vi "Configure Alarm.vi"(8 "error in (no error)":errorcluster, 10 "Alarm Clear Method (0: Safe)":i32(ring) items=["Safe", "Auto"], 11 "VISA resource name":refnum<visa-resource-name>) -> (0 "error out":errorcluster, 3 "VISA resource name out":refnum<visa-resource-name>)   [LabVIEW 2023]
doc: "Configures the method of clearing OHP, FAN, AC-FAIL, and SD alarms."
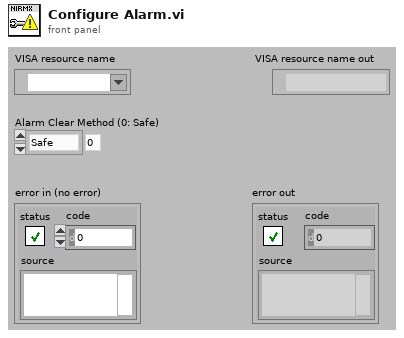
[diagram p1: front panel]
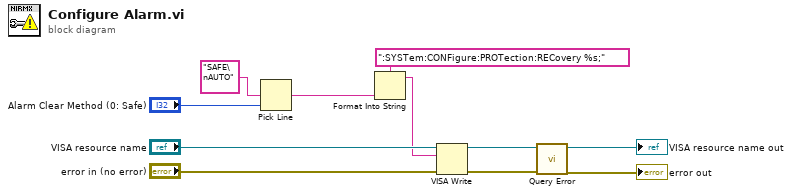
[diagram p0: block diagram]
diagram:
  n1 = Pick Line(multi-line string="SAFE\nAUTO", line index="Alarm Clear Method (0: Safe)") -> (output string=w9:string)  [unwired: 1 in]
  n2 = Format Into String(format string=":SYSTem:CONFigure:PROTection:RECovery %s;", w9) -> (resulting string=w1:string)  [unwired: 2 in, 1 out]
  n3 = VISA Write(VISA resource name="VISA resource name", write buffer=w1, error in (no error)="error in (no error)") -> (VISA resource name out=w5:refnum<visa-resource-name>, error out=w4:errorcluster)  [unwired: 1 out]
  n4 = call "Query Error.vi"("error in (no error)"=w4, "VISA resource name"=w5) -> ("error out"=→"error out":errorcluster, "VISA resource name out"=→"VISA resource name out":refnum<visa-resource-name>)  [unwired: 6 in, 2 out]
